vi "randmatcher.vi"() -> ()   [LabVIEW 2022 SP3]
panel:
  out "Time to match":dbl format="%_5f"
  out "Number Iterations":i32 format="%#.0f"
  out "Current Number":i32 format="%#.0f"
  in  "Number to Match":i32 min=0 max=10000 step=1 format="%#.0f"
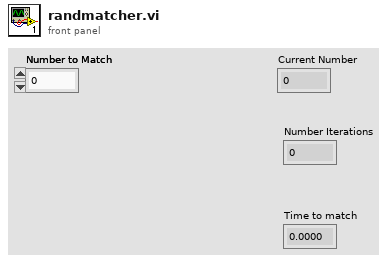
[diagram p1: front panel]
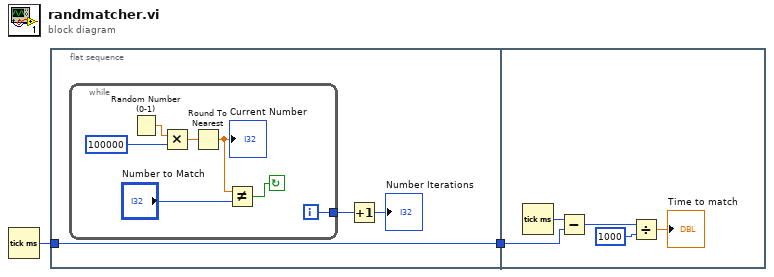
[diagram p0: block diagram]
diagram:
  n1 = Tick Count (ms)() -> (millisecond timer value=w2:u32)
  n2 = flat-sequence {
    tunnel: w2 -> [w3]
    tunnel: [w3] -> w1
    tunnel: w1 -> [w13]
    frame #0 {
      n3 = while {
        tunnel: [w6] -> w5
        i -> [w6]
        stop <- w7 continue-if-true
        n4 = Random Number (0-1)() -> (number: 0 to 1=w12:dbl)
        n5 = Multiply(x=w12, y=100000) -> (x*y=w10:dbl)
        n6 = Round To Nearest(number=w10) -> (nearest integer value=w8:dbl)
        "Current Number" <- w8
        n7 = Not Equal?(x=w8, y="Number to Match") -> (x != y?=w7:bool)
      }
      n8 = Increment(x=w5) -> (x+1=→"Number Iterations":i32)
    }
    frame #1 {
      n9 = Tick Count (ms)() -> (millisecond timer value=w15:u32)
      n10 = Subtract(x=w15, y=w13) -> (x-y=w14:u32)
      n11 = Divide(x=w14, y=1000) -> (x/y=→"Time to match":dbl)
    }
  }
